vi "Draw Line.vi"(6 "Colour":u32(colorbox), 9 "Point 2":T1, 10 "Point 1":T1, 11 "Pixel Data in":u32[][](array[numeric])) -> (3 "Pixel Data out":u32[][](array[numeric]))   [LabVIEW 2020]
uses:
  ce09c930-e75c-45b5-9de7-7d3097d91b09.vi
  8aa8c736-0805-475e-bbf3-9937bbefdeb4.vi
  Point 2D (I32).ctl
  Raster (FPGA).lvlib
panel:
  out "Processing Time [s]":dbl format="%.1p"
  out "Iteration":i32
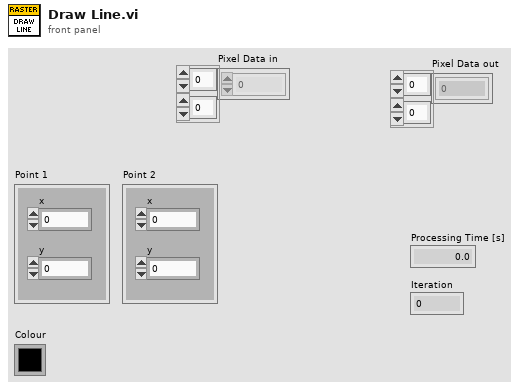
[diagram p1: front panel]
types:
  T1 = typedef "Raster (FPGA).lvlib/Point 2D (I32).ctl" = cluster{"x":i32, "y":i32}
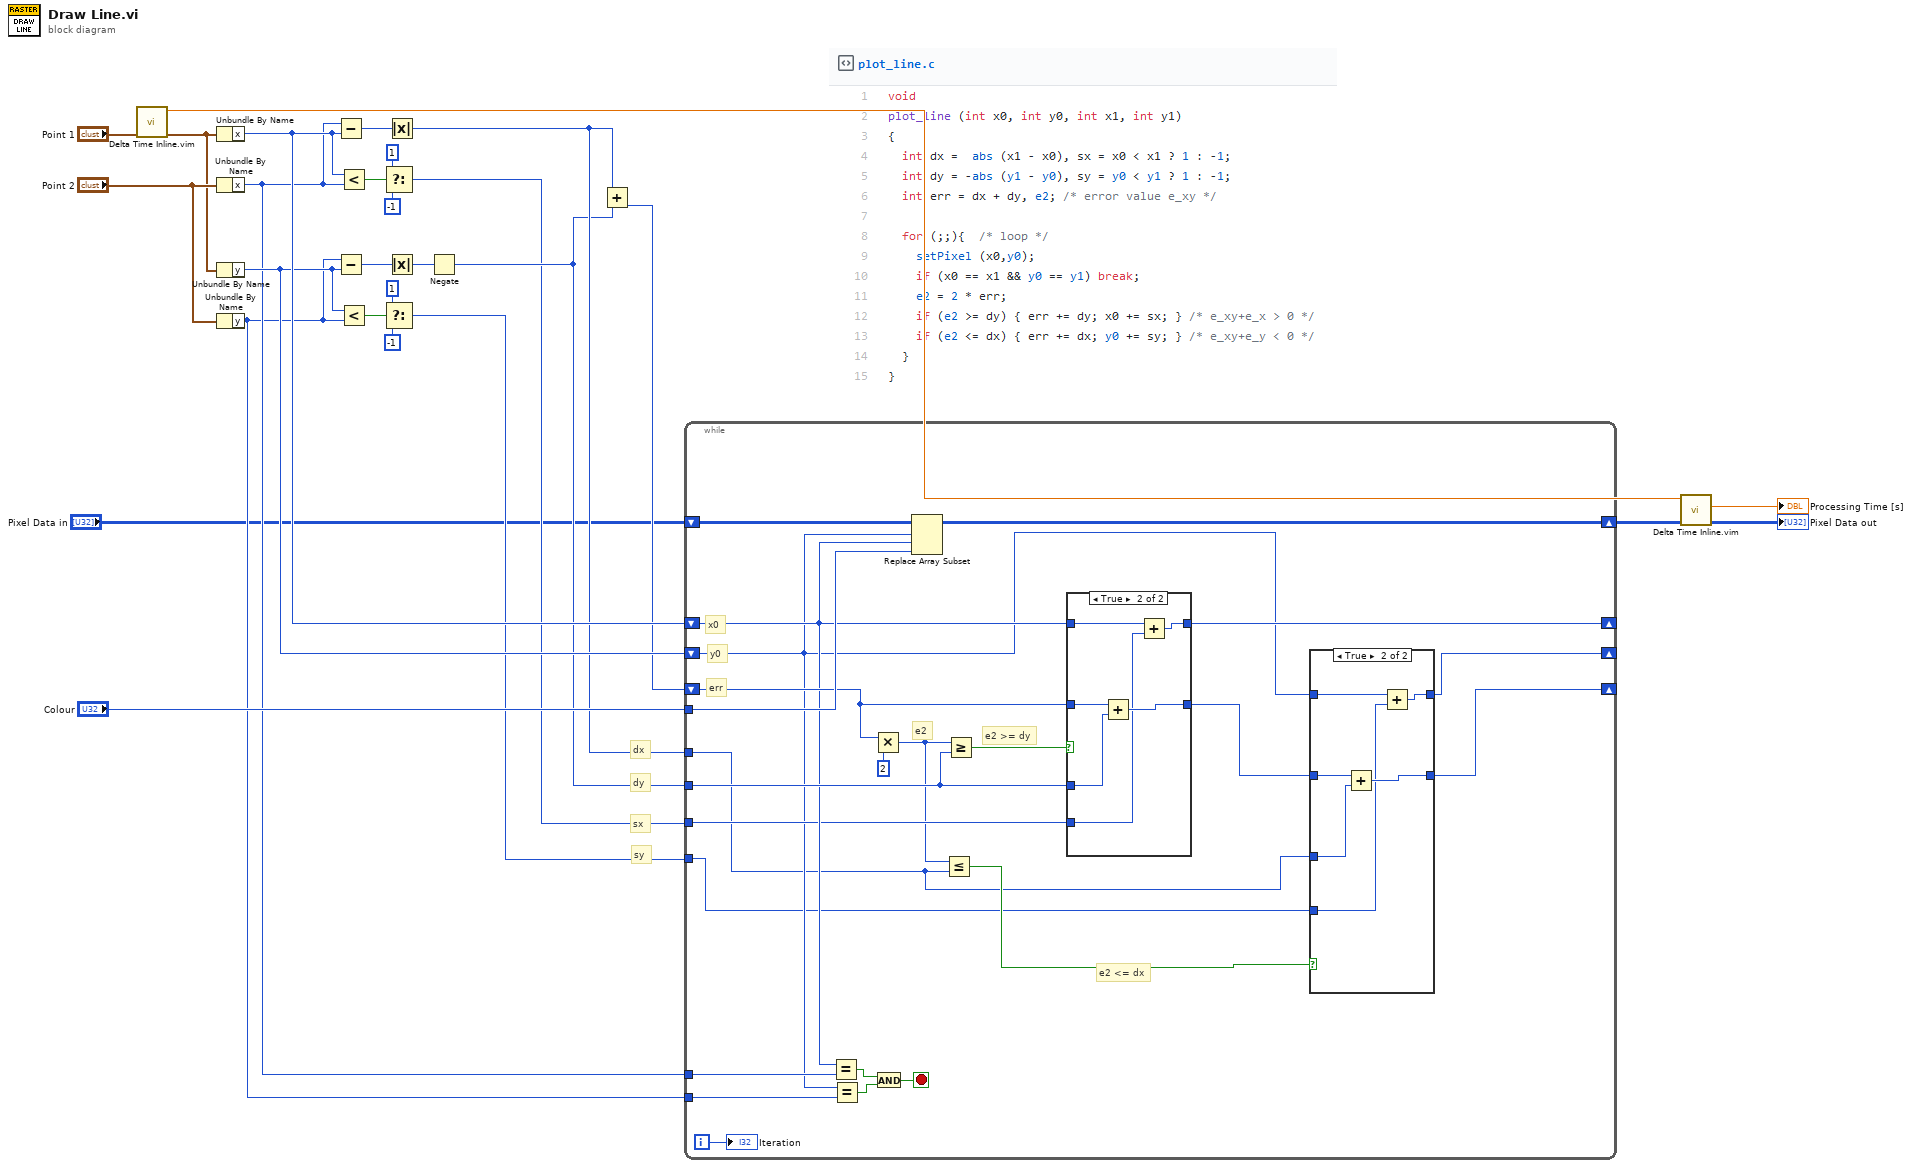
[diagram p0: block diagram]
diagram:
  # "sy"
  # "sx"
  # "dy"
  # "dx"
  n1 = call "Delta Time Inline.vim"("value in"="Point 1") -> ("value out"=w3:T1, "Relative Seconds out [s]"=w2:dbl)  [unwired: 8 in, 1 out]
  n2 = Unbundle By Name(w3) -> ("x"=w17:i32)
  n3 = Unbundle By Name("Point 2") -> ("x"=w14:i32)
  n4 = Unbundle By Name(w3) -> ("y"=w16:i32)
  n5 = Unbundle By Name("Point 2") -> ("y"=w13:i32)
  n6 = Subtract(x=w14, y=w17) -> (x-y=w27:i32)
  n7 = Subtract(x=w13, y=w16) -> (x-y=w20:i32)
  n8 = Less?(x=w17, y=w14) -> (x < y?=w26:bool)
  n9 = Less?(x=w16, y=w13) -> (x < y?=w21:bool)
  n10 = Select(t=1 ("x-y"), s=w26, f=-1 ("x-y")) -> (s? t:f=w9:i32)
  n11 = Select(t=1 ("x-y"), s=w21, f=-1 ("x-y")) -> (s? t:f=w8:i32)
  n12 = Absolute Value(x=w27) -> (abs(x)=w11:i32)
  n13 = Absolute Value(x=w20) -> (abs(x)=w18:i32)
  n14 = Negate(x=w18) -> (-x=w10:i32)
  n15 = Add(x=w11, y=w10) -> (x+y=w12:i32)
  n16 = while {
    shift-right: [w39] -> _
    shift-left: w17 -> [w41]
    shift-right: [w34] -> _
    shift-left: w16 -> [w35]
    tunnel: "Colour" -> [w51]
    tunnel: w14 -> [w50]
    tunnel: w13 -> [w49]
    shift-right: [w32] -> _
    shift-left: w12 -> [w43]
    tunnel: w11 -> [w33]
    tunnel: w10 -> [w42]
    tunnel: w9 -> [w40]
    tunnel: w8 -> [w31]
    shift-right: [w28] -> w7
    shift-left: "Pixel Data in" -> [w29]
    i -> [w30]
    stop <- w46 stop-if-true
    # "e2 <= dx"
    # "e2 >= dy"
    # "e2"
    # "err"
    # "y0"
    # "x0"
    n17 = Equal?(x=w41, y=w50) -> (x = y?=w48:bool)
    n18 = Equal?(x=w35, y=w49) -> (x = y?=w47:bool)
    n19 = Multiply(x=w43, y=2) -> (x*y=w38:i32)
    n20 = And(x=w48, y=w47) -> (x .and. y?=w46:bool)
    n21 = Replace Array Subset(array=w29, new element=w51, index (row)=w35, index (col)=w41) -> (w28:u32[][])
    n22 = Less Or Equal?(x=w38, y=w33) -> (x <= y?=w37:bool)
    n23 = Greater Or Equal?(x=w38, y=w42) -> (x >= y?=w44:bool)
    n24 = case shown="True" w44 {
      tunnel: w43 -> [w52 w59]
      tunnel: w42 -> [_ w58]
      tunnel: [w52 w57] -> w36
      tunnel: w41 -> [w53 w56]
      tunnel: w40 -> [_ w55]
      tunnel: [w53 w54] -> w39
      frame False {
      }
      frame True {
        n25 = Add(x=w59, y=w58) -> (x+y=w57:i32)
        n26 = Add(x=w56, y=w55) -> (x+y=w54:i32)
      }
    }
    n27 = case shown="True" w37 {
      tunnel: w36 -> [w61 w67]
      tunnel: w33 -> [_ w66]
      tunnel: [w61 w65] -> w32
      tunnel: w35 -> [w60 w64]
      tunnel: w31 -> [_ w63]
      tunnel: [w60 w62] -> w34
      frame False {
      }
      frame True {
        n28 = Add(x=w67, y=w66) -> (x+y=w65:i32)
        n29 = Add(x=w64, y=w63) -> (x+y=w62:i32)
      }
    }
    "Iteration" <- w30
  }
  n30 = call "Delta Time Inline.vim"("value in"=w7, "Relative Seconds in [s]"=w2) -> ("value out"=→"Pixel Data out":u32[][], "Delta Time [s]"=→"Processing Time [s]":dbl)  [unwired: 7 in, 1 out]
